vi "Draw_Vanishing.vi"(8 "Draw?":bool=TRUE, 9 "point":cluster{"x":dbl, "y":dbl}, 11 "picture in":picture) -> (1 "right_line":cluster{"slope":dbl, "b":dbl, "theta":dbl}, 2 "left_line":cluster{"slope":dbl, "b":dbl, "theta":dbl}, 3 "picture out":picture)   [LabVIEW 2022 SP3]
uses:
  Perspective_Globals.vi
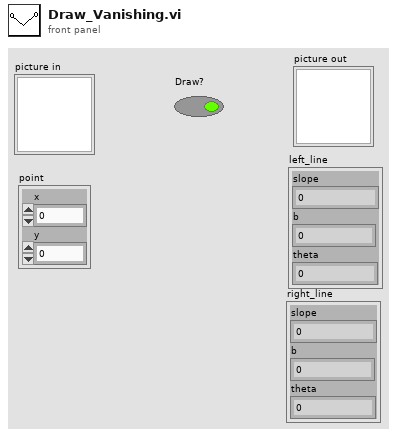
[diagram p1: front panel]
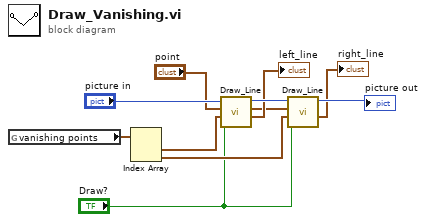
[diagram p0: block diagram]
diagram:
  n1 = global read "Perspective_Globals.vi" "vanishing points"() -> (w2:cluster{"x":dbl, "y":dbl}[])
  n2 = Index Array(array=w2) -> (element #1=w7:cluster{"x":dbl, "y":dbl}, element #2=w6:cluster{"x":dbl, "y":dbl})  [unwired: 2 in]
  n3 = call "Draw_Line.vi"("Draw?"="Draw?", "end"=w7, "start"="point", "picture in"="picture in") -> ("line"=→"left_line":cluster{"slope":dbl, "b":dbl, "theta":dbl}, "picture out"=w9:picture)  [unwired: 6 in]
  n4 = call "Draw_Line.vi"("Draw?"="Draw?", "end"=w6, "start"="point", "picture in"=w9) -> ("line"=→"right_line":cluster{"slope":dbl, "b":dbl, "theta":dbl}, "picture out"=→"picture out":picture)  [unwired: 6 in]
